vi "MH_SetMarkerEnable.vi"(4 "En4":bool=TRUE, 6 "En3":bool=TRUE, 8 "error in (no error)":errorcluster, 9 "En2":bool=TRUE, 10 "En1":bool=TRUE, 11 "devidx":i32) -> (0 "error out":errorcluster, 3 "return type":i32)   [LabVIEW 2019]
uses:
  MH_DllPath_global.vi
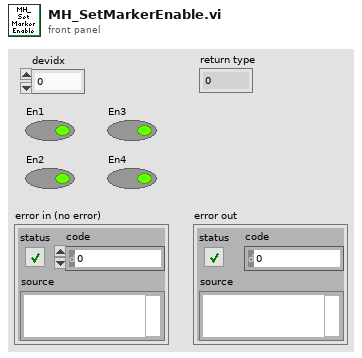
[diagram p1: front panel]
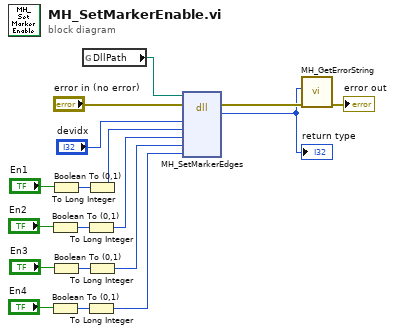
[diagram p0: block diagram]
diagram:
  n1 = Boolean To (0,1)(Boolean="En2") -> (0, 1=w9:i16)
  n2 = Boolean To (0,1)(Boolean="En4") -> (0, 1=w5:i16)
  n3 = Boolean To (0,1)(Boolean="En1") -> (0, 1=w11:i16)
  n4 = Boolean To (0,1)(Boolean="En3") -> (0, 1=w4:i16)
  n5 = global read "MH_DllPath_global.vi" "DllPath"() -> (w17:path)
  n6 = To Long Integer(number=w9) -> (32bit integer=w7:i32)
  n7 = To Long Integer(number=w5) -> (32bit integer=w1:i32)
  n8 = To Long Integer(number=w11) -> (32bit integer=w10:i32)
  n9 = To Long Integer(number=w4) -> (32bit integer=w2:i32)
  n10 = dll-call lib="MHLib64.dll" fn="MH_SetMarkerEdges"(path in=w17, error in="error in (no error)", "devidx"="devidx", "en1"=w10, "en2"=w7, "en3"=w2, "en4"=w1) -> (error out=w15:errorcluster, "return type"=w14:i32)  [unwired: 6 in, 1 out]
  "return type" <- w14
  n11 = call "MH_GetErrorString.vi"("error in (no error)"=w15, "code"=w14) -> ("error out"=→"error out":errorcluster)  [unwired: 7 in, 2 out]
